vi "simpleserver.vi"() -> ()   [LabVIEW 2017]
panel:
  in  "LabView MESSAGE":string
  out "Python MESSAGE":string
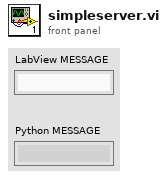
[diagram p1: front panel]
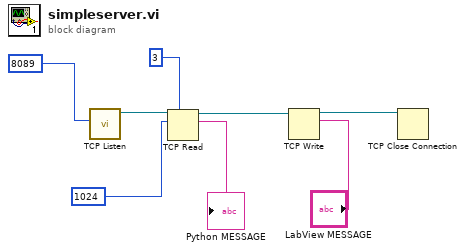
[diagram p0: block diagram]
diagram:
  n1 = call <vilib>:"TCP Listen.vi"("port"=8089) -> ("connection ID"=w7:refnum<k5>)  [unwired: 6 in, 4 out]
  n2 = TCP Read(connection ID=w7, bytes to read=1024, 7:3) -> (connection ID out=w6:refnum<k5>, data out=→"Python MESSAGE":string)  [unwired: 2 in, 1 out]
  n3 = TCP Write(connection ID=w6, data in="LabView MESSAGE") -> (connection ID out=w5:refnum<k5>)  [unwired: 2 in, 2 out]
  n4 = TCP Close Connection(connection ID=w5) -> ()  [unwired: 2 in, 2 out]
